vi "TCP_Server-InputShapes.vi"() -> ()   [LabVIEW 2024]
doc: "This example performs writes and reads on a serial port, as directed by the user. You can press the Write and Read buttons, and change the Read Count, while the example is running.\n\nThe parameters set for the serial port must match the parameters of the connected instrument or device. In this example, the Read Count parameter specifies the number of bytes that the serial port reads. If there were more bytes at the port than the specified number, those bytes would not be read. If there were less bytes at the port than the specified number, you would receive a timeout error.\n\nThis example expands upon the flow control options for XON and XOFF, allowing the user to choose those control characters. Also, the user can enable or disable a termination character. Some devices require a termination character in order to identify the end of command strings. Some devices send a termination character to signify the end of data to be read. This example shows how you can end the Read operation once a termination character is detected in the buffer and/or append a termination character at the end of the Write data."
panel:
  in  "Octagon":bool
  in  "Polygon":bool
  in  "Rectangle":bool
  in  "Line":bool
  out "Numeric 2":u32
  out "data out":string
  out "Numeric":i32
  out "Boolean":bool=TRUE
  in  "Pause":bool=TRUE
  out "Waveform Chart":u32(graph)
  in  "port":u16=3333
  in  "address":string="192.168.210.128"
  in  "Command D":bool
  in  "Command C":bool
  out "error":bool
  out "Connected":bool
  out "Response 2":string
  in  "Command B":bool
  in  "Command A":bool
  in  "Toggle LED":bool
  in  "Enum":T1(ring)
  in  "Stop":bool
  out "Response":string
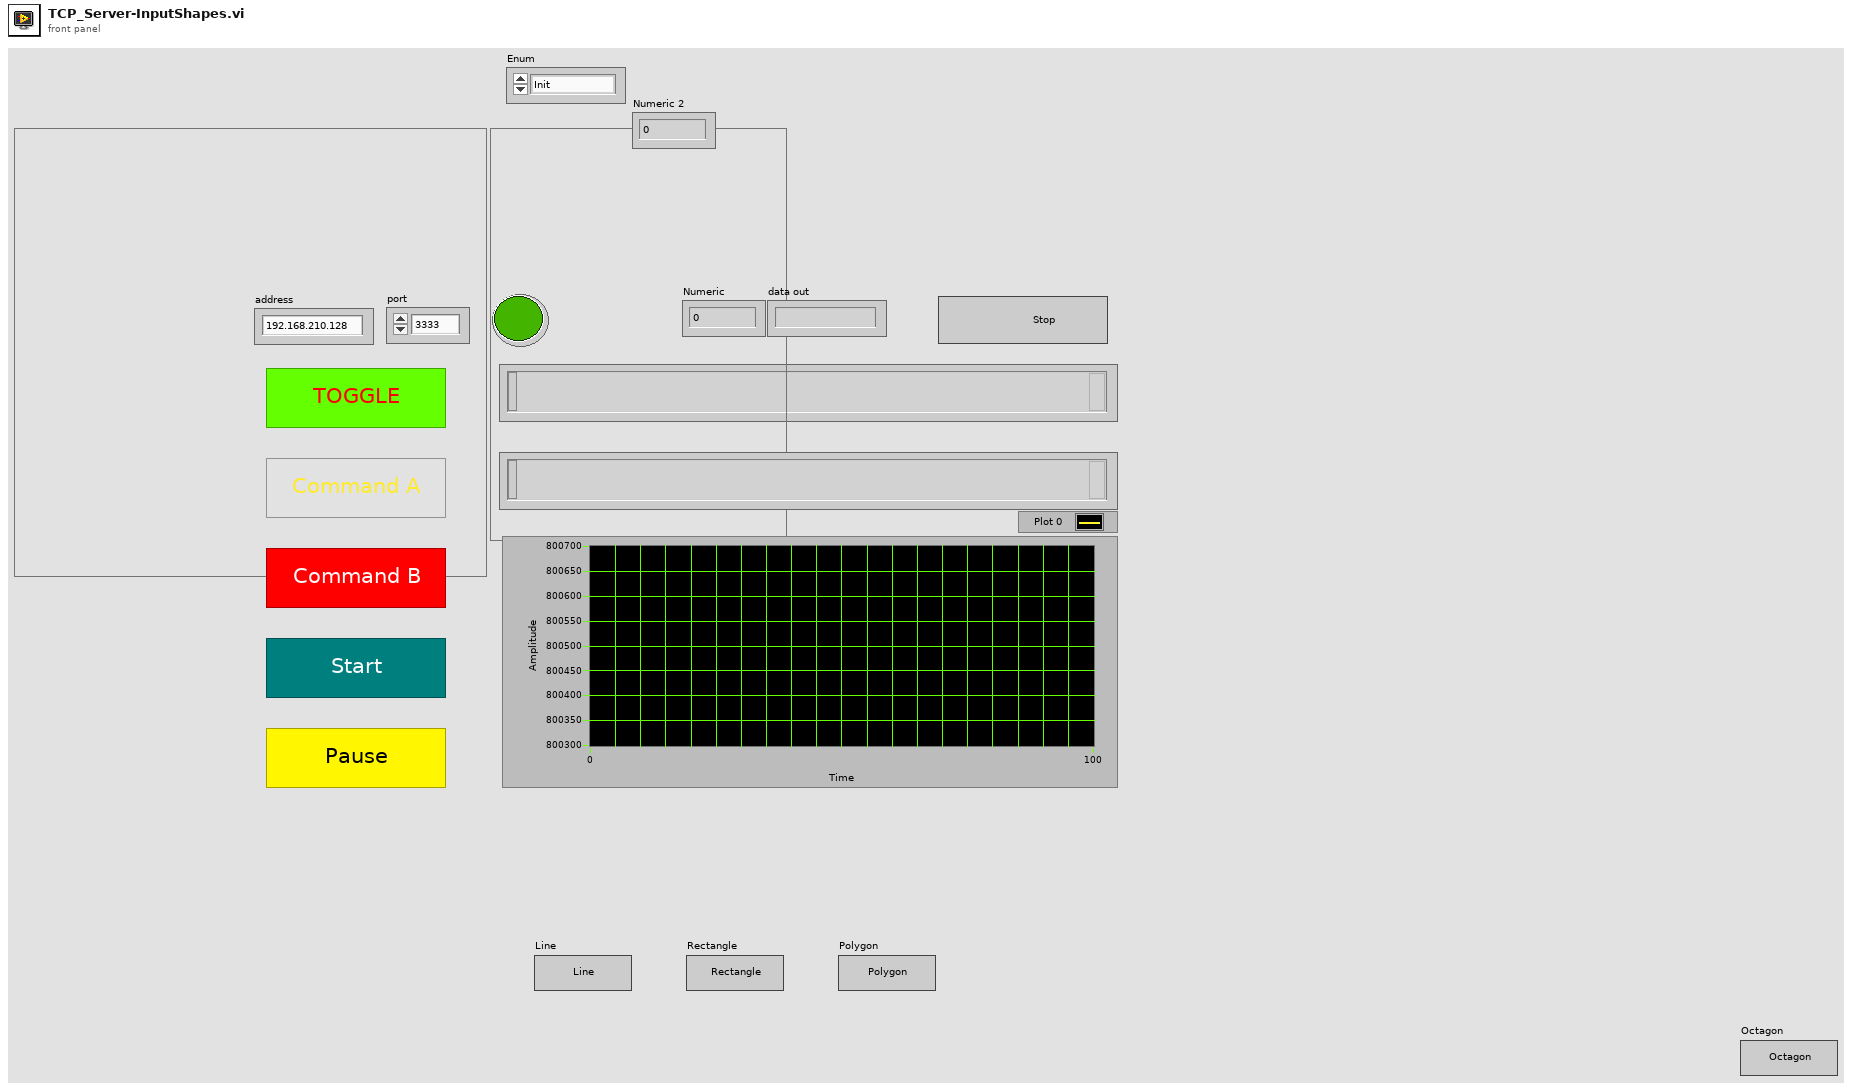
[diagram p1: front panel]
types:
  T1 = enum8{"Init", "Connect", "idle", "send", "wait", "receive", "que", "error", "exit"}
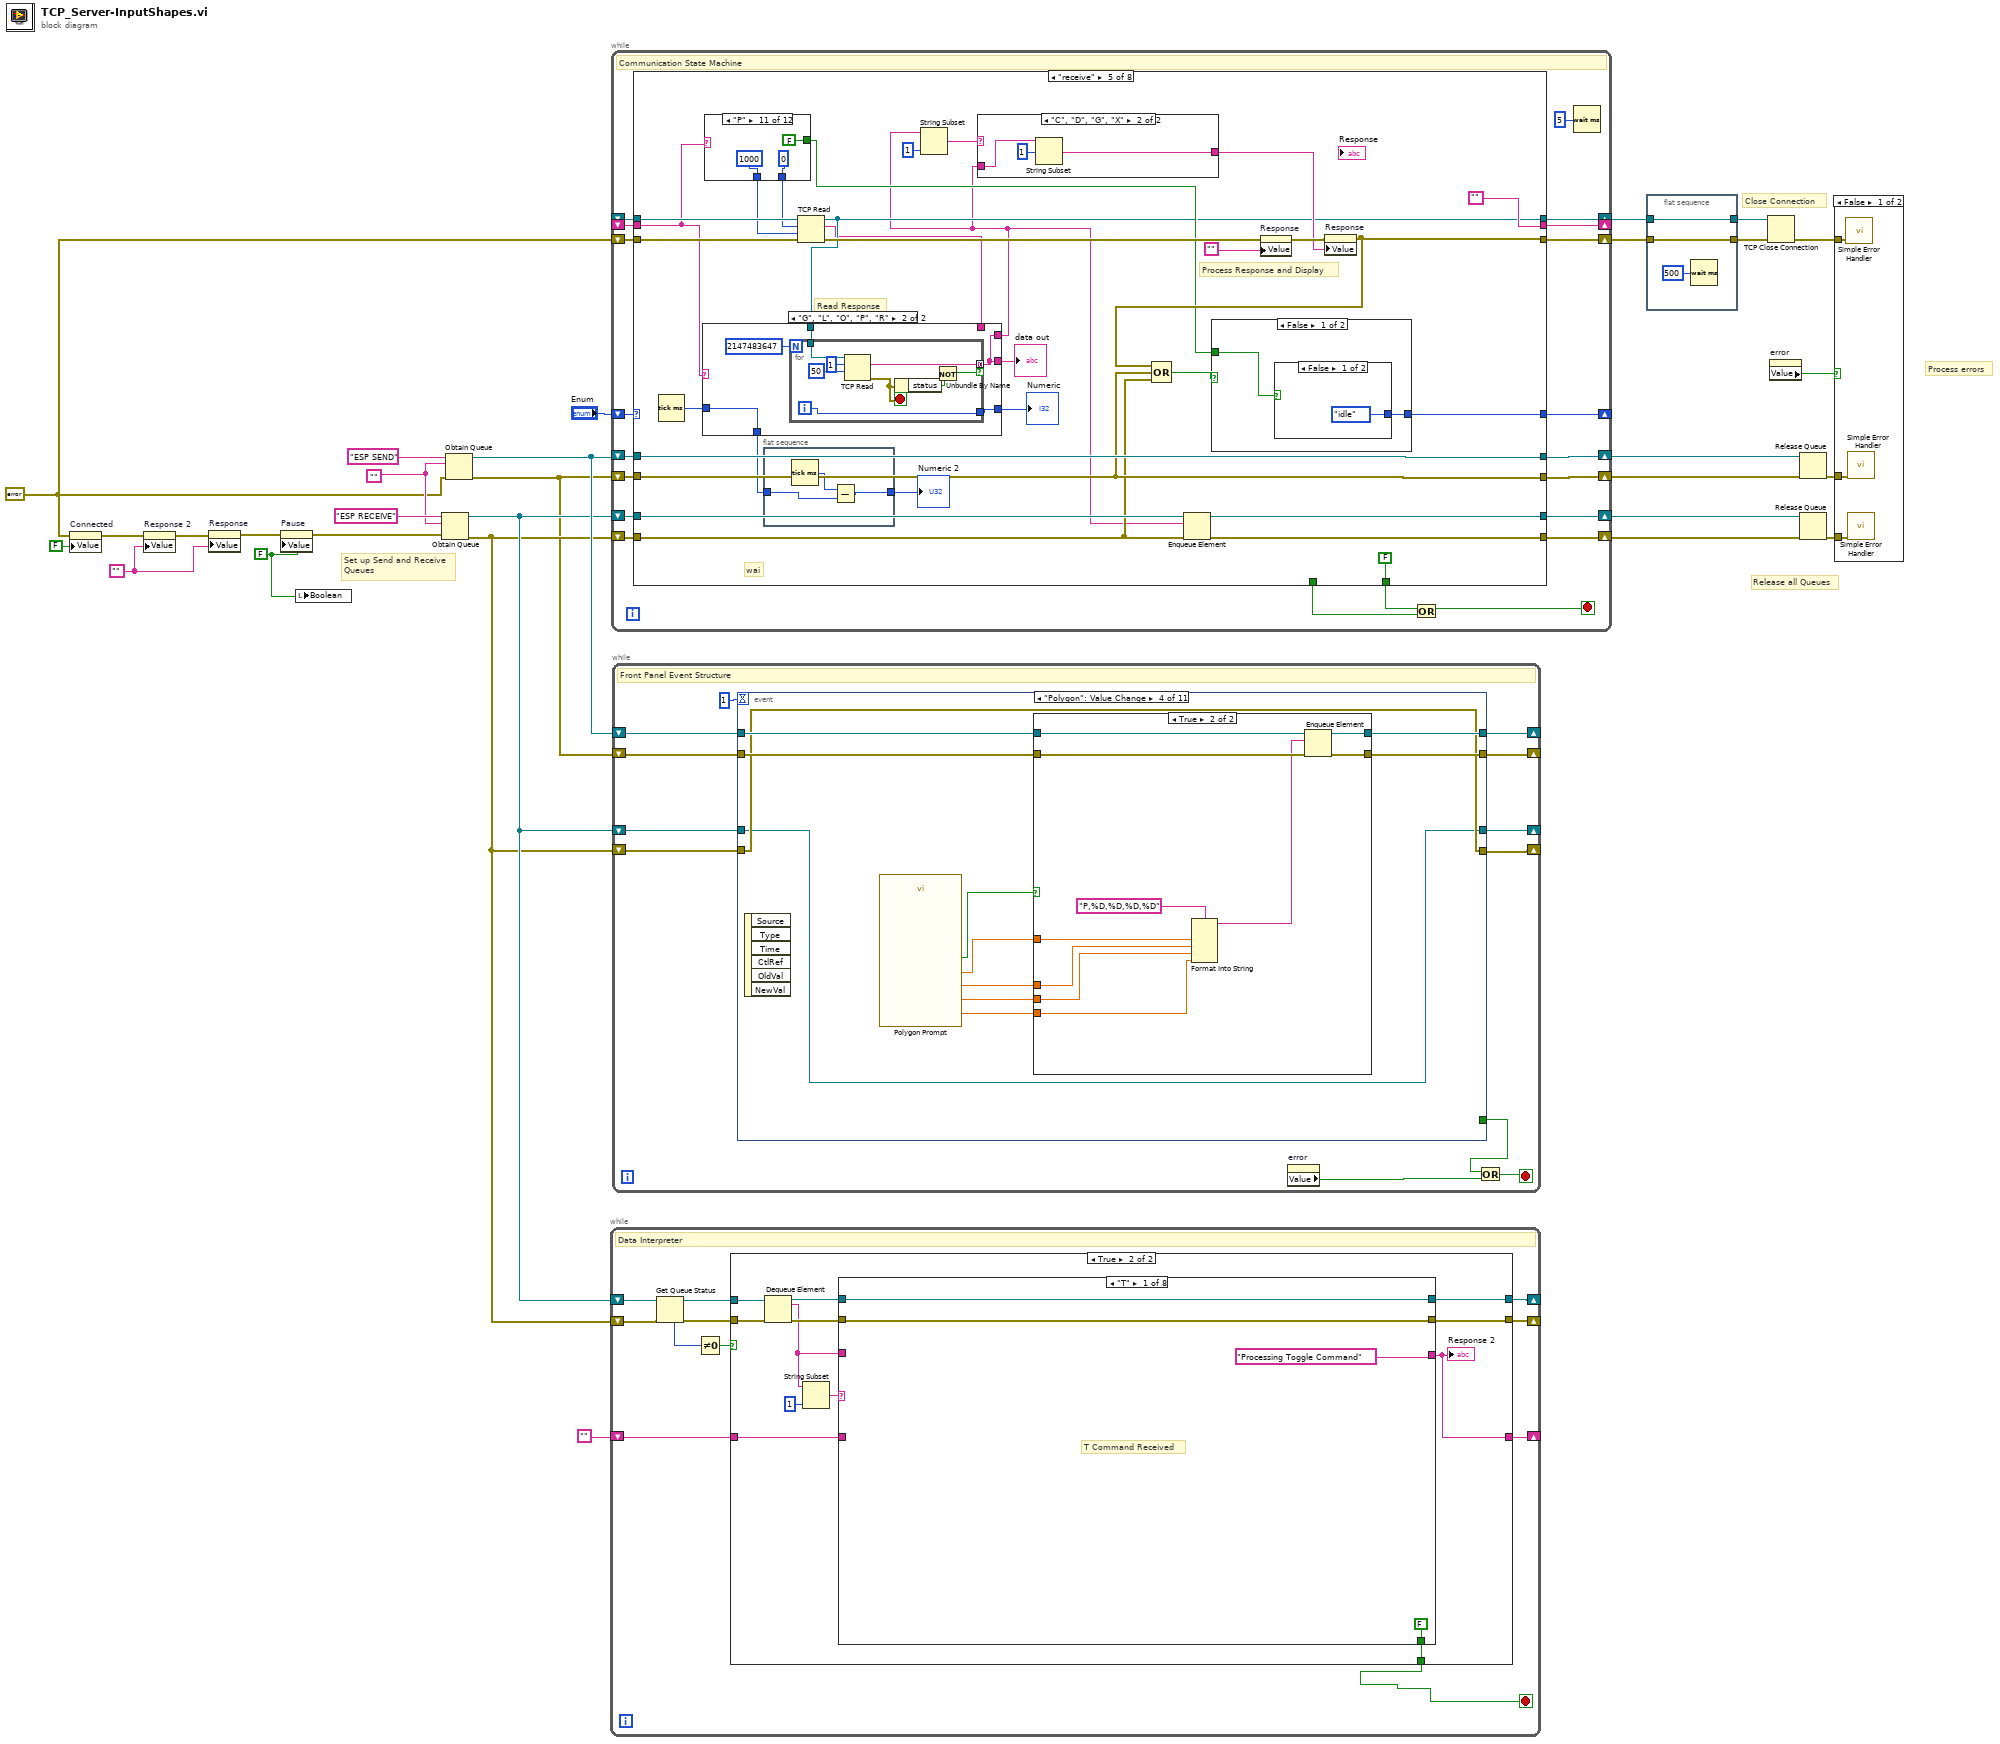
[diagram p0: block diagram]
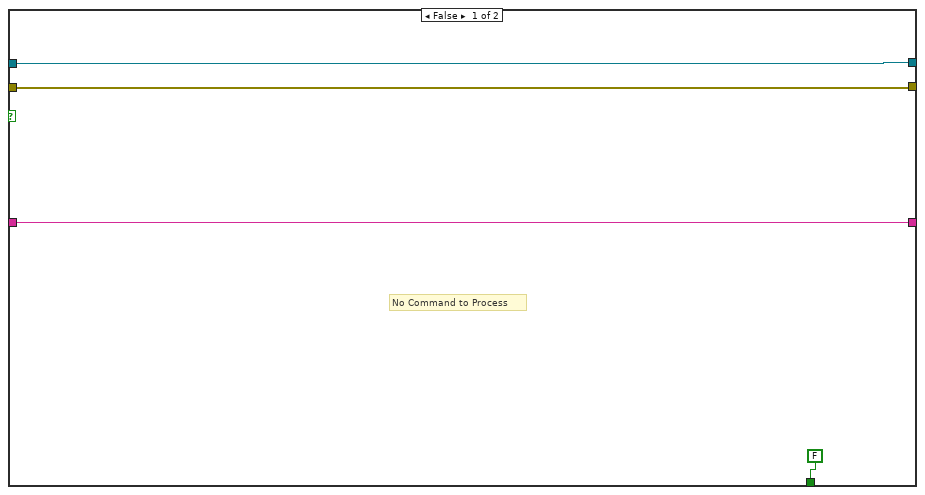
[diagram p3: hidden frame]
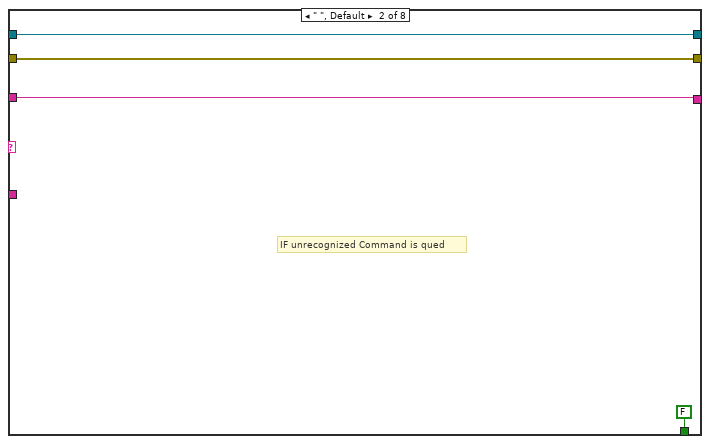
[diagram p4: hidden frame]
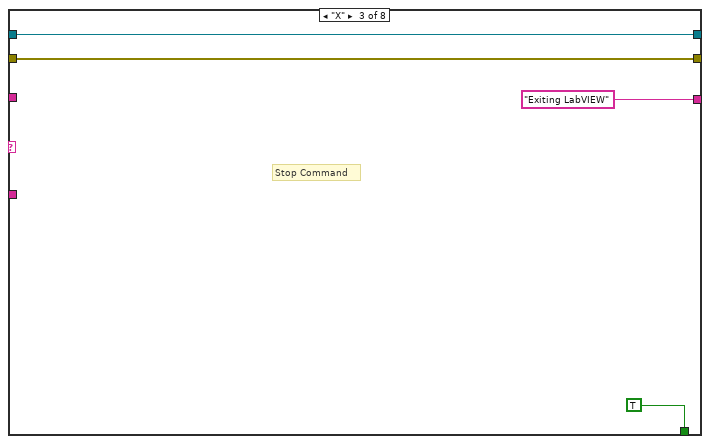
[diagram p5: hidden frame]
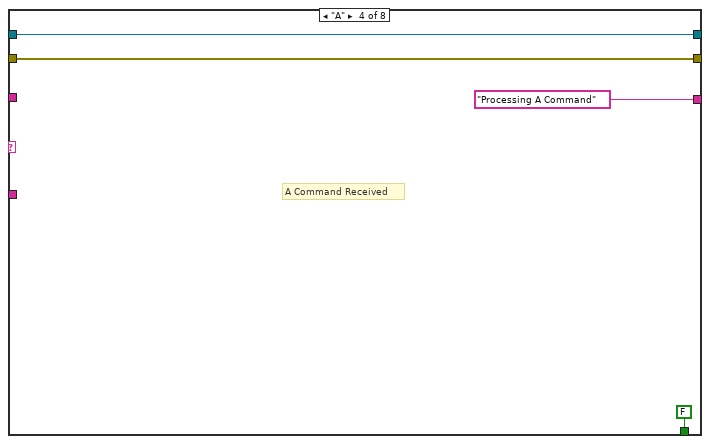
[diagram p6: hidden frame]
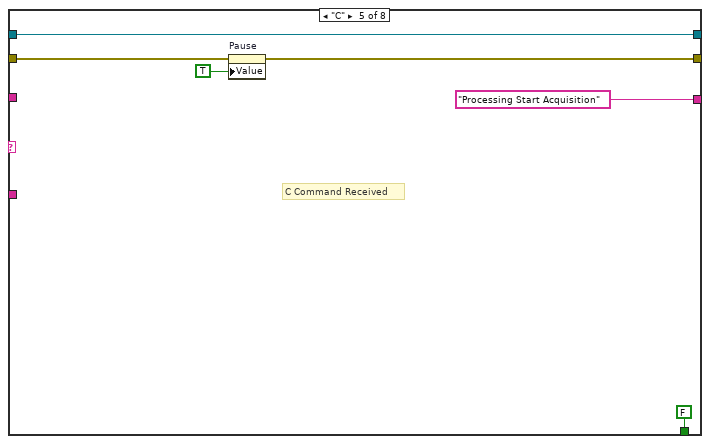
[diagram p7: hidden frame]
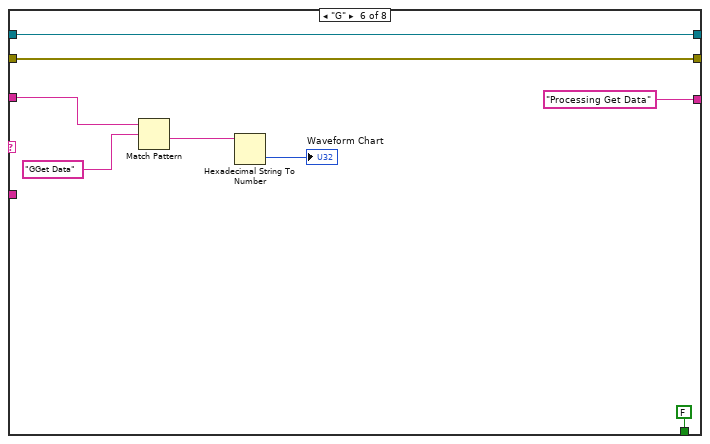
[diagram p8: hidden frame]
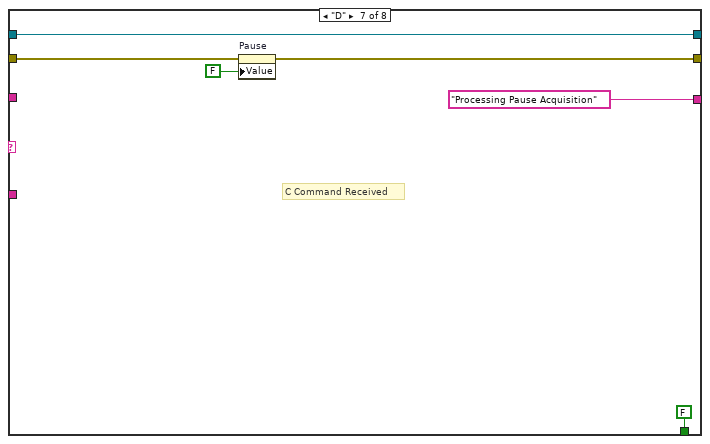
[diagram p9: hidden frame]
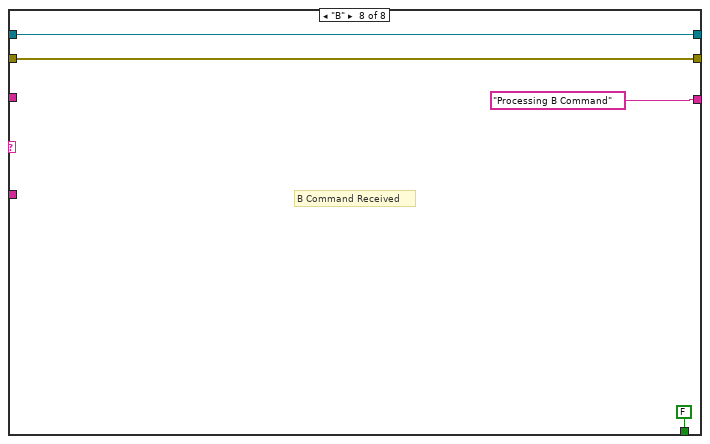
[diagram p10: hidden frame]
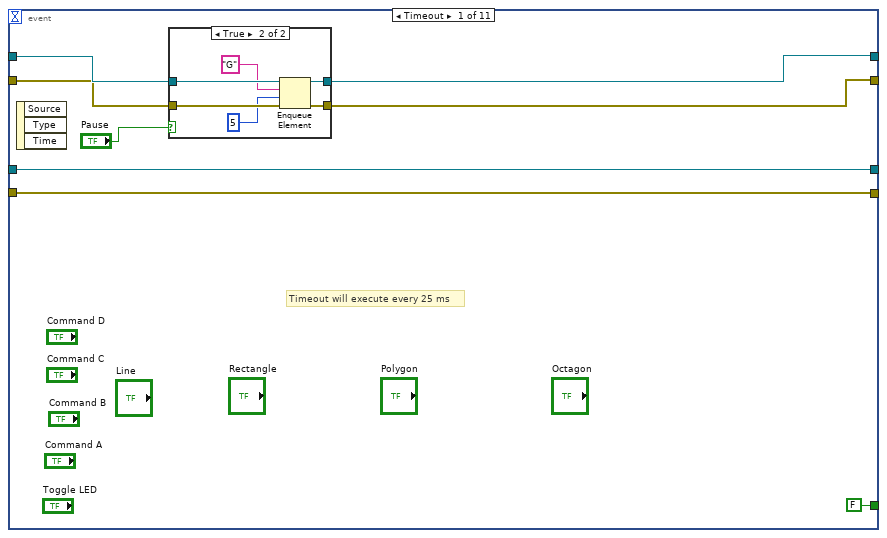
[diagram p11: hidden frame]
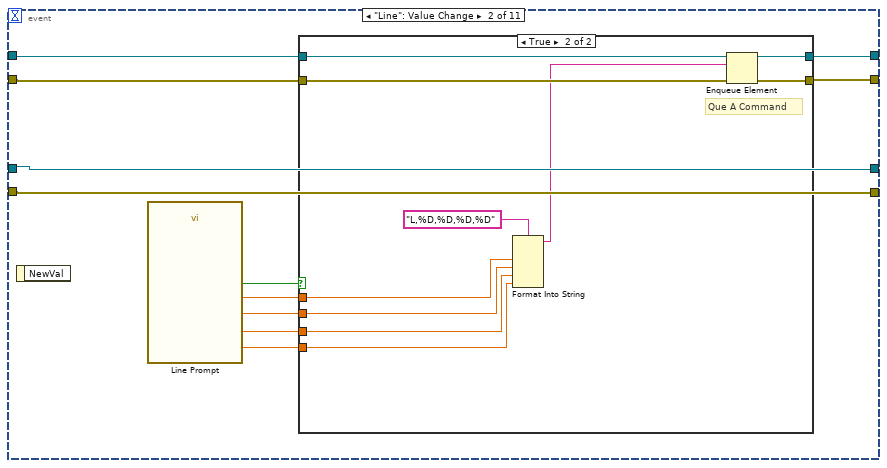
[diagram p13: hidden frame]
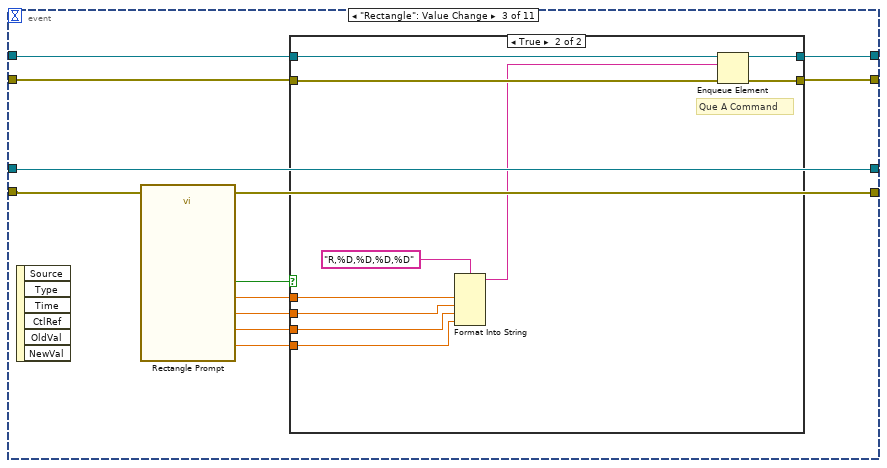
[diagram p15: hidden frame]
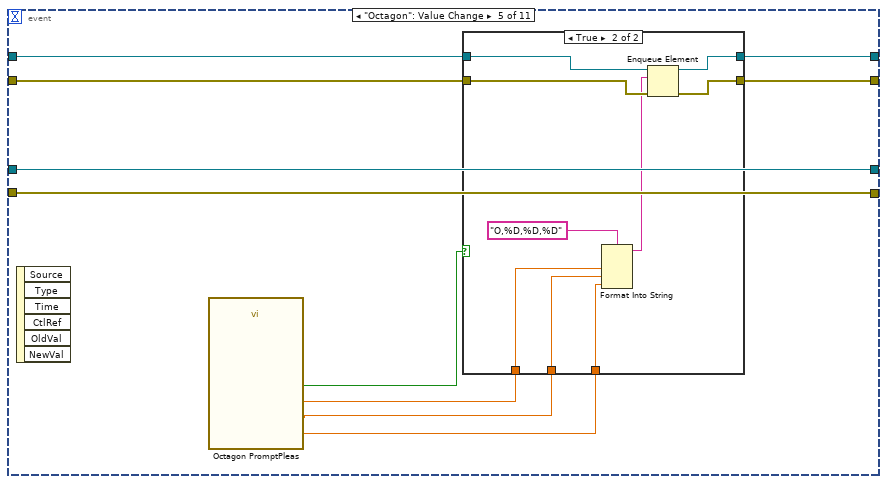
[diagram p18: hidden frame]
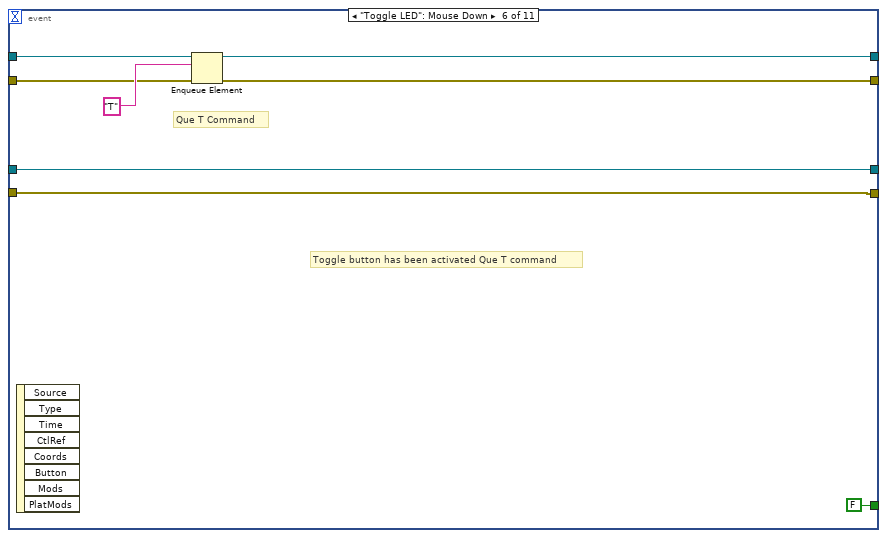
[diagram p20: hidden frame]
diagram:
  w6 = errorcluster {"status"=FALSE, "code"=0, "source"=""} ("error in (no error)")
  w9 = ""
  w5 = FALSE
  w21 = ""
  # "Process errors"
  # "Release all Queues"
  # "Close Connection"
  # "Set up Send and Receive\nQueues"
  n1 = property on="Connected" class="Bool (strict)"(error in=w6, "Value"=FALSE ("Connected")) -> (error out=w8:errorcluster)  [unwired: 1 in, 1 out]
  n2 = property on="Response 2" class="Str"(error in=w8, "Value"=w9) -> (error out=w10:errorcluster)  [unwired: 1 in, 1 out]
  n3 = property on="Response" class="Str"(error in=w10, "Value"=w9) -> (error out=w11:errorcluster)  [unwired: 1 in, 1 out]
  n4 = property on="Pause" class="Bool (strict)"(error in=w11, "Value"=w5) -> (error out=w12:errorcluster)  [unwired: 1 in, 1 out]
  n5 = local write "Boolean"(w5) -> ()
  n6 = Obtain Queue(name (unnamed)="ESP RECEIVE", element data type=w21, error in (no error)=w12) -> (queue out=w20:refnum<queue>, error out=w19:errorcluster)  [unwired: 2 in, 1 out]
  n7 = Obtain Queue(name (unnamed)="ESP SEND", element data type=w21, error in (no error)=w6) -> (queue out=w23:refnum<queue>, error out=w15:errorcluster)  [unwired: 2 in, 1 out]
  n8 = while {
    shift-right: [w34] -> _
    shift-left: w20 -> [w40]
    shift-right: [w33] -> _
    shift-left: w19 -> [w39]
    shift-right: [w32] -> _
    shift-left: "" -> [w31]
    stop <- w30 stop-if-true
    # "Data Interpreter"
    n9 = Get Queue Status(queue=w40, error in (no error)=w39) -> (queue out=w36:refnum<queue>, error out=w35:errorcluster, # elements in queue=w38:i32)  [unwired: 1 in, 5 out]
    n10 = Not Equal To 0?(x=w38) -> (x != 0?=w37:bool)
    n11 = case shown="True" w37 {
      tunnel: w36 -> [w44 w56]
      tunnel: w35 -> [w43 w55]
      tunnel: [w44 w50] -> w34
      tunnel: [w43 w49] -> w33
      tunnel: [FALSE w48] -> w30
      tunnel: [w41 w46] -> w32
      tunnel: w31 -> [w41 w45]
      frame False {
        # "No Command to Process"
      }
      frame True {
        n12 = Dequeue Element(queue=w56, error in (no error)=w55) -> (queue out=w54:refnum<queue>, element=w47:string, error out=w53:errorcluster)  [unwired: 1 in, 1 out]
        n13 = String Subset(string=w47, length (rest)=1 ("length (rest)")) -> (substring=w51:string)  [unwired: 1 in]
        n14 = case shown="\"T\"" w51 {
          tunnel: w54 -> [w60 w64 w68 w72 w78 w84 w92 w96]
          tunnel: w53 -> [w59 w63 w67 w71 w75 w85 w89 w95]
          tunnel: [w60 w64 w68 w72 w78 w84 w92 w96] -> w50
          tunnel: [w59 w63 w67 w71 w73 w85 w87 w95] -> w49
          tunnel: w47 -> [_ w61 _ _ _ w81 _ _]
          tunnel: [FALSE FALSE TRUE FALSE FALSE FALSE FALSE FALSE] -> w48
          tunnel: ["Processing Toggle Command" w61 "Exiting LabVIEW" "Processing A Command" "Processing Start Acquisition" "Processing Get Data" "Processing Pause Acquisition" "Processing B Command"] -> w46
          tunnel: w45 -> [_ _ _ _ _ _ _ _]
          frame "T" {
            # "T Command Received"
          }
          frame " ", Default {
            # "IF unrecognized Command is qued"
          }
          frame "X" {
            # "Stop Command"
          }
          frame "A" {
            # "A Command Received"
          }
          frame "C" {
            # "C Command Received"
            n15 = property on="Pause" class="Bool (strict)"(error in=w75, "Value"=TRUE ("Value (Signaling)")) -> (error out=w73:errorcluster)  [unwired: 1 in, 1 out]
          }
          frame "G" {
            n16 = Match Pattern(string=w81, regular expression="GGet Data") -> (after substring=w80:string)  [unwired: 1 in, 3 out]
            n17 = Hexadecimal String To Number(string=w80) -> (number=→"Waveform Chart":u32)  [unwired: 2 in, 1 out]
          }
          frame "D" {
            # "C Command Received"
            n18 = property on="Pause" class="Bool (strict)"(error in=w89, "Value"=FALSE ("Value (Signaling)")) -> (error out=w87:errorcluster)  [unwired: 1 in, 1 out]
          }
          frame "B" {
            # "B Command Received"
          }
        }
        "Response 2" <- w46
      }
    }
  }
  n19 = while {
    shift-right: [w108] -> w29
    shift-left: w23 -> [w116]
    shift-right: [w107] -> w27
    shift-left: w15 -> [w115]
    shift-right: [w106] -> w28
    shift-left: w20 -> [w114]
    shift-right: [w105] -> w24
    shift-left: w19 -> [w113]
    shift-right: [w103] -> _
    shift-left: "Enum" -> [w102]
    shift-right: [w112] -> w4
    shift-left: _ -> [w109]
    shift-right: [w111] -> w3
    shift-left: w6 -> [w110]
    shift-right: [w101] -> _
    shift-left: _ -> [w100]
    stop <- w98 stop-if-true
    # "Communication State Machine"
    n20 = case shown="\"receive\"" w102 {
      selector: w102 -> [_ _ _ _ _ _ w313 _]
      tunnel: [w132 w147 w173 w186 w222 w296 w312 w338] -> w108
      tunnel: [w127 w142 w170 w183 w217 w293 w311 w337] -> w107
      tunnel: [w131 w145 w171 w187 w223 T1."exit" ("Enum") w313 T1."idle" ("Enum")] -> w103
      tunnel: w116 -> [w132 w149 w175 w186 w222 w296 w312 w338]
      tunnel: w115 -> [w127 w148 w174 w183 w217 w293 w311 w337]
      tunnel: w114 -> [w133 w143 w172 w185 w221 w295 w310 w336]
      tunnel: w113 -> [w126 w141 w169 w182 w216 w292 w301 w335]
      tunnel: [w121 w138 w158 w180 w201 w297 w315 w319] -> w112
      tunnel: [w120 w137 w159 w179 w218 w294 w314 w320] -> w111
      tunnel: w110 -> [w119 w137 w163 w179 w213 w294 w314 w330]
      tunnel: w109 -> [_ w138 w164 w180 w212 w297 w315 w329]
      tunnel: [w133 w143 w172 w185 w219 w295 w308 w336] -> w106
      tunnel: [w126 w141 w169 w182 w220 w292 w304 w335] -> w105
      tunnel: [FALSE FALSE FALSE FALSE FALSE FALSE TRUE FALSE] -> w99
      tunnel: ["" "" w157 w178 "" "" "" ""] -> w101
      tunnel: w100 -> [_ _ _ w178 w200 _ _ _]
      tunnel: [_ _ _ _ _ _ "Stop" _] -> w97
      frame "Init", Default {
        # "Init State ::  Connect to Internet via WiFi"
        n21 = property on="error" class="Bool (strict)"("Value"=FALSE ("error")) -> ()  [unwired: 2 in, 2 out]
        n22 = property on="Response 2" class="Str"("Value"="") -> ()  [unwired: 2 in, 2 out]
        n23 = TCP Open Connection(address="address", remote port or service name="port", timeout ms (60000)=60000, error in (no error)=w119) -> (connection ID=w121:refnum<k5>, error out=w120:errorcluster)  [unwired: 1 in]
        n24 = Or(x=w126, y=w127) -> (x .or. y?=w128:bool)
        n25 = Or(x=w120, y=w128) -> (x .or. y?=w129:bool)
        n26 = case shown="False" w129 {
          tunnel: [T1."Connect" ("Enum") T1."error" ("Enum")] -> w131
          frame False {
          }
          frame True {
          }
        }
      }
      frame "idle" {
        # "Wait until Command is in queue"
        n27 = Get Queue Status(queue=w149, error in (no error)=w148) -> (queue out=w147:refnum<queue>, error out=w142:errorcluster, # elements in queue=w146:i32)  [unwired: 1 in, 5 out]
        n28 = Not Equal To 0?(x=w146) -> (x != 0?=w144:bool)
        n29 = Compound Arithmetic op=OR(w137, w142, w141) -> (w140:bool)
        n30 = case shown="False" w140 {
          tunnel: [w151 T1."error" ("Enum")] -> w145
          tunnel: w144 -> [w150 _]
          frame False {
            n31 = case shown="True" w150 {
              tunnel: [T1."idle" ("Enum") T1."send" ("Enum")] -> w151
              frame False {
              }
              frame True {
              }
            }
          }
          frame True {
          }
        }
      }
      frame "send" {
        # "Read and Discard Echo Command"
        # "Send Command"
        n32 = Dequeue Element(queue=w175, error in (no error)=w174) -> (queue out=w173:refnum<queue>, element=w165:string, error out=w170:errorcluster)  [unwired: 1 in, 1 out]
        n33 = Concatenate Strings(w165, "\r\n") -> (w162:string)
        n34 = TCP Write(connection ID=w164, data in=w162, error in (no error)=w163) -> (connection ID out=w160:refnum<k5>, error out=w161:errorcluster)  [unwired: 2 out]
        n35 = TCP Read(connection ID=w160, bytes to read=1, error in (no error)=w161, 9:5000 ("timeout ms (25000)")) -> (connection ID out=w158:refnum<k5>, data out=w157:string, error out=w159:errorcluster)  [unwired: 1 out]
        n36 = Compound Arithmetic op=OR(w159, w170, w169) -> (w168:bool)
        n37 = case shown="False" w168 {
          tunnel: [T1."wait" ("Enum") T1."error" ("Enum")] -> w171
          frame False {
          }
          frame True {
          }
        }
      }
      frame "wait" {
        # "Wait for actual Response"
        n38 = Compound Arithmetic op=OR(w179, w183, w182) -> (w184:bool)
        n39 = case shown="False" w184 {
          tunnel: [w189 T1."error" ("Enum")] -> w187
          frame False {
            n40 = case shown="True" TRUE {
              tunnel: [T1."wait" ("Enum") T1."receive" ("Enum")] -> w189
              frame False {
              }
              frame True {
              }
            }
          }
          frame True {
          }
        }
      }
      frame "receive" {
        # "wai"
        # "Process Response and Display"
        # "Read Response"
        n41 = Tick Count (ms)() -> (millisecond timer value=w195:u32)
        n42 = case shown="\"P\"" w200 {
          tunnel: [25 16 25 20 20 22 0 0 0 0 0 21] -> w208
          tunnel: [10 ("timeout ms (25000)") 10 ("timeout ms (25000)") 10 ("timeout ms (25000)") 10 ("timeout ms (25000)") 10 ("timeout ms (25000)") 10 ("timeout ms (25000)") 1000 ("timeout ms (25000)") 1000 ("timeout ms (25000)") 1000 ("timeout ms (25000)") 1000 ("timeout ms (25000)") 1000 ("timeout ms (25000)") 10 ("timeout ms (25000)")] -> w207
          tunnel: [FALSE TRUE FALSE FALSE FALSE FALSE FALSE FALSE FALSE FALSE FALSE FALSE] -> w202
          frame "False", Default {
          }
          frame "X" {
          }
          frame "T" {
          }
          frame "A" {
          }
          frame "B" {
          }
          frame "C" {
          }
          frame "G" {
          }
          frame "L" {
          }
          frame "R" {
          }
          frame "O" {
          }
          frame "P" {
          }
          frame "D" {
          }
        }
        n43 = flat-sequence {
          tunnel: w194 -> [w225]
          tunnel: [w224] -> w193
          frame #0 {
            n44 = Tick Count (ms)() -> (millisecond timer value=w226:u32)
            n45 = Subtract(x=w226, y=w225) -> (x-y=w224:u32)
          }
        }
        n46 = TCP Read(connection ID=w212, bytes to read=w208, error in (no error)=w213, 9:w207) -> (connection ID out=w201:refnum<k5>, data out=w197:string, error out=w211:errorcluster)  [unwired: 1 in]
        n47 = case shown="\"G\", \"L\", \"O\", \"P\", \"R\"" w200 {
          tunnel: w201 -> [_ w233]
          tunnel: [_ w231] -> w199
          tunnel: [_ w230] -> w198
          tunnel: w197 -> [w228 _]
          tunnel: [w228 w230] -> w196
          tunnel: w195 -> [w227 w229]
          tunnel: [w227 w229] -> w194
          frame "False", Default {
          }
          frame "G", "L", "O", "P", "R" {
            n48 = for {
              N: 2147483647 -> [_]
              tunnel: w233 -> [w241]
              tunnel: [w238] -> w230 mode=concatenating if=w235
              tunnel: [w234] -> w231
              i -> [w234]
              stop <- w237 stop-if-true
              n49 = TCP Read(connection ID=w241, bytes to read=1, 9:50 ("timeout ms (25000)")) -> (data out=w238:string, error out=w237:errorcluster)  [unwired: 2 in, 1 out]
              n50 = Unbundle By Name(w237) -> ("status"=w236:bool)
              n51 = Not(x=w236) -> (.not. x?=w235:bool)
            }
          }
        }
        "Numeric" <- w199
        "data out" <- w198
        n52 = String Subset(string=w196, length (rest)=1 ("length (rest)")) -> (substring=w205:string)  [unwired: 1 in]
        n53 = case shown="\"C\", \"D\", \"G\", \"X\"" w205 {
          tunnel: w196 -> [w242 w244]
          tunnel: [w242 w243] -> w204
          frame "False", Default {
          }
          frame "C", "D", "G", "X" {
            n54 = String Subset(string=w244, offset (0)=1) -> (substring=w243:string)  [unwired: 1 in]
          }
        }
        n55 = Enqueue Element(queue=w221, element=w196, error in (no error)=w216) -> (queue out=w219:refnum<queue>, error out=w220:errorcluster)  [unwired: 1 in, 1 out]
        n56 = property on="Response" class="Str"(error in=w211, "Value"="") -> (error out=w209:errorcluster)  [unwired: 1 in, 1 out]
        n57 = property on="Response" class="Str"(error in=w209, "Value"=w204) -> (error out=w218:errorcluster)  [unwired: 1 in, 1 out]
        n58 = Compound Arithmetic op=OR(w218, w217, w216) -> (w215:bool)
        n59 = case shown="False" w215 {
          tunnel: [w283 T1."error" ("Enum")] -> w223
          tunnel: w202 -> [w282 _]
          frame False {
            n60 = case shown="False" w282 {
              tunnel: [T1."idle" ("Enum") T1."exit" ("Enum")] -> w283
              frame False {
              }
              frame True {
              }
            }
          }
          frame True {
          }
        }
        "Numeric 2" <- w193
      }
      frame "error" {
        # "Process any error"
        n61 = Build Array(w294, w293, w292) -> (w291:errorcluster[])
        n62 = for {
          tunnel: w291 -> [w298] mode=indexing
          n63 = call <vilib>:"General Error Handler.vi"("error in (no error)"=w298) -> ()  [unwired: 10 in, 5 out]
        }
        "error" <- TRUE ("error")
      }
      frame "exit" {
        # "Exit due to error"
        n64 = Enqueue Element(queue=w310, element="D", error in (no error)=w301) -> (queue out=w308:refnum<queue>, error out=w306:errorcluster)  [unwired: 1 in, 1 out]
        n65 = property on="Connected" class="Bool (strict)"(error in=w306, "Value"=FALSE ("Connected")) -> (error out=w305:errorcluster)  [unwired: 1 in, 1 out]
        n66 = property on="Response" class="Str"(error in=w305, "Value"="") -> (error out=w304:errorcluster)  [unwired: 1 in, 1 out]
      }
      frame "Connect" {
        # "Validating connection"
        # "Send ID to validate connection"
        # "Clear any residual characters"
        n67 = Concatenate Strings("I" ("write buffer"), "\r\n") -> (w328:string)
        n68 = TCP Write(connection ID=w329, data in=w328, error in (no error)=w330) -> (connection ID out=w327:refnum<k5>, error out=w326:errorcluster)  [unwired: 2 out]
        n69 = flat-sequence {
          tunnel: w327 -> [w340]
          tunnel: [w340] -> w325
          frame #0 {
            n70 = Wait (ms)(milliseconds to wait=u32 5) -> ()  [unwired: 1 out]
          }
        }
        n71 = TCP Read(connection ID=w325, bytes to read=8, error in (no error)=w326) -> (connection ID out=w319:refnum<k5>, data out=w318:string, error out=w320:errorcluster)  [unwired: 2 out]
        n72 = Search/Split String(string=w318, search string/char (-)="IESP32") -> (match + rest of string=w323:string)  [unwired: 1 in, 2 out]
        n73 = String Length(string=w323) -> (length=w322:i32)
        n74 = Not Equal To 0?(x=w322) -> (x != 0?=→"Connected":bool)
      }
    }
    n75 = Or(x=w99, y=w97) -> (x .or. y?=w98:bool)
    n76 = Wait (ms)(milliseconds to wait=u32 5) -> ()  [unwired: 1 out]
  }
  n77 = while {
    shift-right: [w349] -> _
    shift-left: w23 -> [w350]
    shift-right: [w348] -> _
    shift-left: w15 -> [w351]
    shift-right: [w344] -> _
    shift-left: w20 -> [w347]
    shift-right: [w345] -> _
    shift-left: w19 -> [w346]
    stop <- w342 stop-if-true
    # "Front Panel Event Structure"
    n78 = event shown="[3] \"Polygon\": Value Change" {
      selector: _ -> [_ _ _ _ _ _ _ _ _ _ _]
      dyn-events: _ -> [_ _ _ _ _ _ _ _ _ _ _]
      timeout: 1 -> [_ _ _ _ _ _ _ _ _ _ _]
      tunnel: w351 -> [w356 w372 w393 w422 w442 w464 w472 w481 w489 w498 w508]
      tunnel: w350 -> [w357 w371 w392 w421 w443 w466 w474 w483 w491 w500 w507]
      tunnel: [w354 w374 w395 w424 w445 w463 w471 w480 w488 w497 w505] -> w349
      tunnel: [w355 w373 w394 w423 w444 w462 w470 w479 w487 w496 w506] -> w348
      tunnel: [FALSE _ _ _ _ FALSE FALSE FALSE FALSE FALSE w501] -> w343
      tunnel: w347 -> [w359 w370 w401 w415 w446 w460 w468 w477 w485 w494 w503]
      tunnel: w346 -> [w358 w369 w402 w416 w447 w459 w467 w476 w484 w493 w502]
      tunnel: [w358 w369 w402 w416 w447 w459 w467 w476 w484 w493 w510] -> w345
      tunnel: [w359 w370 w401 w415 w446 w460 w468 w477 w485 w494 w503] -> w344
      event Timeout {
        # "Timeout will execute every 25 ms"
        n79 = event-data() -> ()  [unwired: 1 in, 3 out]
        n80 = case shown="True" "Pause" {
          tunnel: w357 -> [w362 w368]
          tunnel: w356 -> [w361 w367]
          tunnel: [w361 w366] -> w355
          tunnel: [w362 w365] -> w354
          frame False {
          }
          frame True {
            n81 = Enqueue Element(queue=w368, element="G", timeout in ms (-1)=5, error in (no error)=w367) -> (queue out=w365:refnum<queue>, error out=w366:errorcluster)  [unwired: 1 out]
          }
        }
      }
      event "Line": Value Change {
        n82 = event-data() -> ()  [unwired: 1 in, 1 out]
        n83 = call "Line Prompt"() -> ("End Point Y"=w376:dbl, "End Point X"=w375:dbl, "Start Point Y"=w377:dbl, "Start Point X"=w378:dbl, "OK"=w379:bool)  [unwired: 14 in, 1 out]
        n84 = case shown="True" w379 {
          tunnel: w371 -> [w381 w391]
          tunnel: w372 -> [w380 w390]
          tunnel: [w381 w389] -> w374
          tunnel: [w380 w388] -> w373
          tunnel: w378 -> [_ w383]
          tunnel: w377 -> [_ w384]
          tunnel: w376 -> [_ w386]
          tunnel: w375 -> [_ w385]
          frame False {
          }
          frame True {
            # "Que A Command"
            n85 = Format Into String(format string="L,%D,%D,%D,%D", w383, w384, w385, w386) -> (resulting string=w382:string)  [unwired: 2 in, 1 out]
            n86 = Enqueue Element(queue=w391, element=w382, error in (no error)=w390) -> (queue out=w389:refnum<queue>, error out=w388:errorcluster)  [unwired: 1 in, 1 out]
          }
        }
      }
      event "Rectangle": Value Change {
        n87 = event-data() -> ()  [unwired: 1 in, 6 out]
        n88 = call "Rectangle Prompt"() -> ("Width"=w396:dbl, "Length"=w397:dbl, "Start Y"=w398:dbl, "Start X"=w399:dbl, "OK"=w400:bool)  [unwired: 14 in, 1 out]
        n89 = case shown="True" w400 {
          tunnel: w392 -> [w404 w414]
          tunnel: w393 -> [w403 w413]
          tunnel: [w404 w412] -> w395
          tunnel: [w403 w411] -> w394
          tunnel: w399 -> [_ w410]
          tunnel: w398 -> [_ w406]
          tunnel: w397 -> [_ w407]
          tunnel: w396 -> [_ w408]
          frame False {
          }
          frame True {
            # "Que A Command"
            n90 = Format Into String(format string="R,%D,%D,%D,%D", w410, w406, w407, w408) -> (resulting string=w405:string)  [unwired: 2 in, 1 out]
            n91 = Enqueue Element(queue=w414, element=w405, error in (no error)=w413) -> (queue out=w412:refnum<queue>, error out=w411:errorcluster)  [unwired: 1 in, 1 out]
          }
        }
      }
      event "Polygon": Value Change {
        n92 = event-data() -> ()  [unwired: 1 in, 6 out]
        n93 = call "Polygon Prompt"() -> ("No of Sides"=w420:dbl, "Radius"=w419:dbl, "Center Y"=w418:dbl, "Center X"=w417:dbl, "OK"=w425:bool)  [unwired: 14 in, 1 out]
        n94 = case shown="True" w425 {
          tunnel: [w427 w437] -> w424
          tunnel: [w426 w436] -> w423
          tunnel: w422 -> [w426 w435]
          tunnel: w421 -> [w427 w434]
          tunnel: w420 -> [_ w431]
          tunnel: w419 -> [_ w430]
          tunnel: w418 -> [_ w429]
          tunnel: w417 -> [_ w428]
          frame False {
          }
          frame True {
            n95 = Format Into String(format string="P,%D,%D,%D,%D", w428, w429, w430, w431) -> (resulting string=w432:string)  [unwired: 2 in, 1 out]
            n96 = Enqueue Element(queue=w434, element=w432, error in (no error)=w435) -> (queue out=w437:refnum<queue>, error out=w436:errorcluster)  [unwired: 1 in, 1 out]
          }
        }
      }
      event "Octagon": Value Change {
        n97 = event-data() -> ()  [unwired: 1 in, 6 out]
        n98 = call "Octagon PromptPleas"() -> ("Radius"=w440:dbl, "Center Y"=w439:dbl, "Center X"=w438:dbl, "OK"=w441:bool)  [unwired: 15 in, 1 out]
        n99 = case shown="True" w441 {
          tunnel: [w449 w458] -> w445
          tunnel: [w448 w457] -> w444
          tunnel: w443 -> [w449 w456]
          tunnel: w442 -> [w448 w455]
          tunnel: w440 -> [_ w453]
          tunnel: w439 -> [_ w452]
          tunnel: w438 -> [_ w451]
          frame False {
          }
          frame True {
            n100 = Format Into String(format string="O,%D,%D,%D", w451, w452, w453) -> (resulting string=w450:string)  [unwired: 2 in, 1 out]
            n101 = Enqueue Element(queue=w456, element=w450, error in (no error)=w455) -> (queue out=w458:refnum<queue>, error out=w457:errorcluster)  [unwired: 1 in, 1 out]
          }
        }
      }
      event "Toggle LED": Mouse Down {
        # "Que T Command"
        # "Toggle button has been activated Que T command"
        n102 = event-data() -> ()  [unwired: 1 in, 8 out]
        n103 = Enqueue Element(queue=w466, element="T", error in (no error)=w464) -> (queue out=w463:refnum<queue>, error out=w462:errorcluster)  [unwired: 1 in, 1 out]
      }
      event "Command A": Mouse Down {
        # "Que A Command"
        # "A Command button has been activated Que A command"
        n104 = event-data() -> ()  [unwired: 1 in, 8 out]
        n105 = Enqueue Element(queue=w474, element="A", error in (no error)=w472) -> (queue out=w471:refnum<queue>, error out=w470:errorcluster)  [unwired: 1 in, 1 out]
      }
      event "Command D": Mouse Down {
        # "Que A Command"
        # "A Command button has been activated Que A command"
        n106 = event-data() -> ()  [unwired: 1 in, 8 out]
        n107 = local write "Pause"(FALSE ("Pause")) -> ()
        n108 = Enqueue Element(queue=w483, element="D", error in (no error)=w481) -> (queue out=w480:refnum<queue>, error out=w479:errorcluster)  [unwired: 1 in, 1 out]
      }
      event "Command B": Mouse Down {
        # "Que B Command"
        # "B Command button has been activated Que B command"
        n109 = event-data() -> ()  [unwired: 1 in, 8 out]
        n110 = Enqueue Element(queue=w491, element="B", error in (no error)=w489) -> (queue out=w488:refnum<queue>, error out=w487:errorcluster)  [unwired: 1 in, 1 out]
      }
      event "Command C": Mouse Down {
        # "Que C Command"
        # "C Command button has been activated Que C command"
        n111 = event-data() -> ()  [unwired: 1 in, 8 out]
        n112 = local write "Pause"(TRUE ("Pause")) -> ()
        n113 = Enqueue Element(queue=w500, element="C", error in (no error)=w498) -> (queue out=w497:refnum<queue>, error out=w496:errorcluster)  [unwired: 1 in, 1 out]
      }
      event "Stop": Value Change {
        w501 = TRUE
        # "Stop Application"
        n114 = event-data() -> ()  [unwired: 1 in, 6 out]
        n115 = Enqueue Element(queue=w507, element="X", error in (no error)=w508) -> (queue out=w505:refnum<queue>, error out=w506:errorcluster)  [unwired: 1 in, 1 out]
        n116 = property on="Connected" class="Bool (strict)"(error in=w502, "Value"=FALSE ("Connected")) -> (error out=w511:errorcluster)  [unwired: 1 in, 1 out]
        n117 = property on="Response" class="Str"(error in=w511, "Value"="") -> (error out=w510:errorcluster)  [unwired: 1 in, 1 out]
        "Boolean" <- w501
      }
    }
    n118 = property on="error" class="Bool (strict)"() -> ("Value"=w341:bool)  [unwired: 2 in, 2 out]
    n119 = Or(x=w343, y=w341) -> (x .or. y?=w342:bool)
  }
  n120 = flat-sequence {
    tunnel: w4 -> [w514]
    tunnel: w3 -> [w515]
    tunnel: [w515] -> w2
    tunnel: [w514] -> w1
    frame #0 {
      n121 = Wait (ms)(milliseconds to wait=u32 500) -> ()  [unwired: 1 out]
    }
  }
  n122 = TCP Close Connection(connection ID=w1, error in (no error)=w2) -> (error out=w13:errorcluster)  [unwired: 2 out]
  n123 = property on="error" class="Bool (strict)"() -> ("Value"=w14:bool)  [unwired: 2 in, 2 out]
  n124 = Release Queue(queue=w29, error in (no error)=w27) -> (error out=w17:errorcluster)  [unwired: 1 in, 2 out]
  n125 = Release Queue(queue=w28, error in (no error)=w24) -> (error out=w16:errorcluster)  [unwired: 1 in, 2 out]
  n126 = case shown="False" w14 {
    tunnel: w13 -> [w518 _]
    tunnel: w17 -> [w517 _]
    tunnel: w16 -> [w516 _]
    frame False {
      n127 = call <vilib>:"Simple Error Handler.vi"("error in (no error)"=w518) -> ()  [unwired: 1 in, 8 out]
      n128 = call <vilib>:"Simple Error Handler.vi"("error in (no error)"=w517) -> ()  [unwired: 1 in, 8 out]
      n129 = call <vilib>:"Simple Error Handler.vi"("error in (no error)"=w516) -> ()  [unwired: 1 in, 8 out]
    }
    frame True {
    }
  }
